vi "AddTestMethod_CreateNewWizard_IncludeItem.vi"(11 "Wizard":T1) -> (3 "Include me":bool)   [LabVIEW 2013]
uses:
  <resource>/Framework/Providers/API/ItemRef.ctl
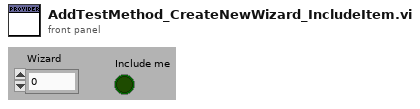
[diagram p1: front panel]
types:
  T1 = typedef "ItemRef.ctl" = u64
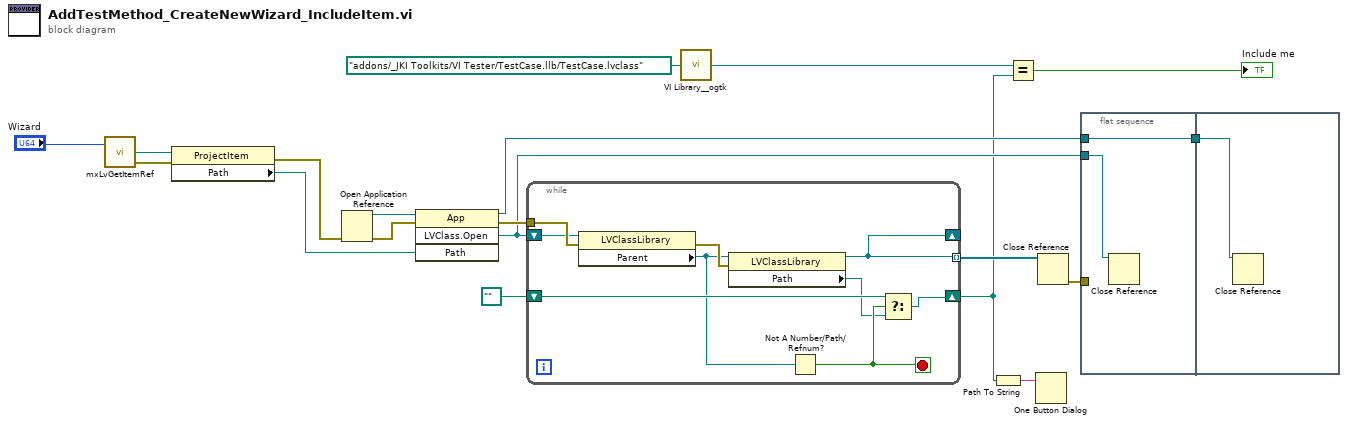
[diagram p0: block diagram]
diagram:
  n1 = call <resource>:"mxLvGetItemRef.vi"("Item"="Wizard") -> ("Item Refnum"=w18:refnum<vi>, "error out"=w15:errorcluster)  [unwired: 1 in, 1 out]
  n2 = property class="ProjectItem"(reference=w18, error in=w15) -> (error out=w14:errorcluster, "Path"=w16:path)  [unwired: 1 out]
  n3 = Open Application Reference(8:w14) -> (0:w13:errorcluster, 3:w17:refnum<vi>)  [unwired: 3 in]
  n4 = invoke class="App" method="LVClass.Open"(reference=w17, error in=w13, "Path"=w16) -> (reference out=w8:refnum<vi>, error out=w12:errorcluster, "LVClass.Open"=w9:refnum<vi>)  [unwired: 1 in, 1 out]
  n5 = while {
    tunnel: w12 -> [w28]
    shift-right: [w21] -> _
    shift-left: w9 -> [w26]
    shift-right: [w22] -> w2
    shift-left: path "" ("Path") -> [w24]
    tunnel: [w21] -> w10 mode=indexing
    stop <- w25 stop-if-true
    n6 = property class="LVClassLibrary"(reference=w26, error in=w28) -> (error out=w27:errorcluster, "Parent"=w20:refnum<vi>)  [unwired: 1 out]
    n7 = property class="LVClassLibrary"(reference=w20, error in=w27) -> (reference out=w21:refnum<vi>, "Path"=w23:path)  [unwired: 1 out]
    n8 = Not A Number/Path/Refnum?(number/path/refnum=w20) -> (NaN/Path/Refnum?=w25:bool)
    n9 = Select(t=w24, s=w25, f=w23) -> (s? t:f=w22:path)
  }
  n10 = call <userlib>:"VI Library__ogtk.vi"("Relative path (.)"=path "addons/_JKI Toolkits/VI Tester/TestCase.llb/TestCase.lvclass") -> ("VI Library (+ Relative)"=w4:path)
  n11 = Path To String(path=w2) -> (string=w1:string)
  n12 = Equal?(x=w4, y=w2) -> (x = y?=→"Include me":bool)
  n13 = One Button Dialog(message=w1) -> ()  [unwired: 1 in, 1 out]
  n14 = Close Reference(reference=w10) -> (error out=w5:errorcluster)  [unwired: 1 in]
  n15 = flat-sequence {
    tunnel: w9 -> [w30]
    tunnel: w8 -> [w29]
    tunnel: [w29] -> w7
    tunnel: w5 -> [_]
    tunnel: w7 -> [w31]
    frame #0 {
      n16 = Close Reference(reference=w30) -> ()  [unwired: 1 in, 1 out]
    }
    frame #1 {
      n17 = Close Reference(reference=w31) -> ()  [unwired: 1 in, 1 out]
    }
  }
